vi "SignalAcqStatus.vi"(8 "error in (no error)":errorcluster caption="entrée d'erreur (pas d'erreur)", 10 "Booléen":bool=TRUE, 11 "Experiment en entrée":refnum<class "Experiment.lvclass"> caption="DNL_LabVIEW Object in") -> (0 "error out":errorcluster caption="sortie d'erreur", 3 "Experiment en sortie":refnum<class "Experiment.lvclass"> caption="DNL_LabVIEW Object out")   [LabVIEW 2019, in "Experiment.lvclass"]
uses:
  Experiment.lvclass
  Experiment.lvclass/Experiment.ctl
  <userlib>/GenProg/ArrayTo1DI32.vi
  DevicesClass/BaseDevice/BaseDevice.lvclass
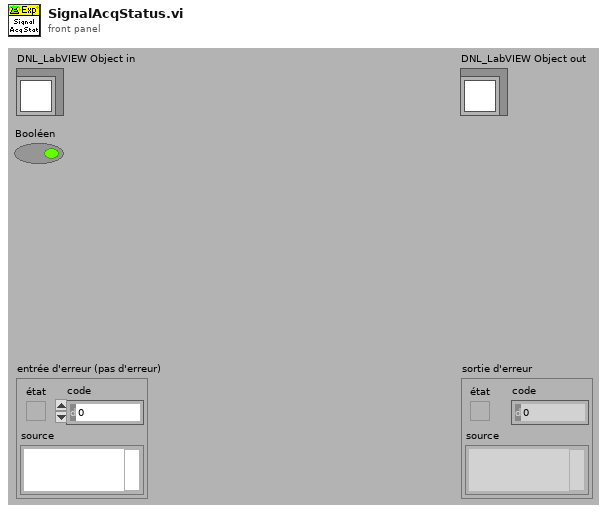
[diagram p1: front panel]
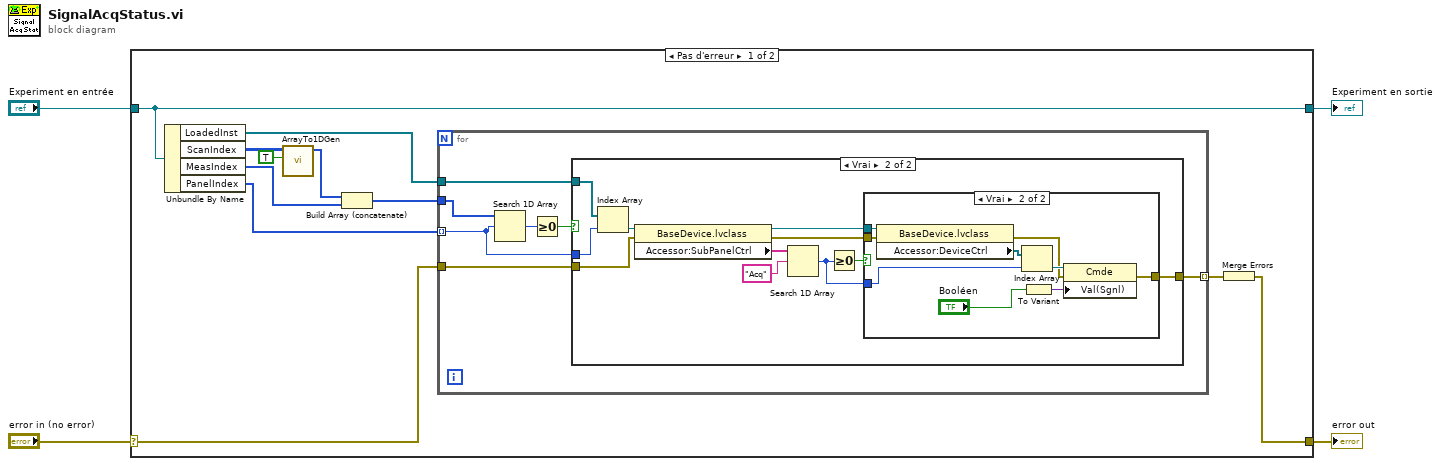
[diagram p0: block diagram]
diagram:
  n1 = case shown="Pas d'erreur" "error in (no error)" {
    selector: "error in (no error)" -> [w7 w46]
    tunnel: [w5 w46] -> w3
    tunnel: [w15 w45] -> w1
    tunnel: "Experiment en entrée" -> [w15 w45]
    frame No Error {
      n2 = Unbundle By Name(w15) -> ("LoadedInst"=w14:refnum<class "BaseDevice.lvclass">[], "ScanIndex"=w13:i32[][], "MeasIndex"=w11:i32[], "PanelIndex"=w8:i32[])
      n3 = call-poly <userlib>:"ArrayTo1DGen.vi"("DelArrEnd"=TRUE, "tableau"=w13) -> ("Array Out"=w10:i32[])  [unwired: 7 in, 2 out]
      n4 = Build Array (concatenate)(w10, w11) -> (w9:i32[])
      n5 = for {
        tunnel: w14 -> [w19]
        tunnel: w9 -> [w22]
        tunnel: w8 -> [w18] mode=indexing
        tunnel: w7 -> [w17]
        tunnel: [w16] -> w6 mode=indexing
        n6 = Search 1D Array(1D array=w22, element=w18) -> (index of element=w21:i32)  [unwired: 1 in]
        n7 = Greater Or Equal To 0?(x=w21) -> (x >= 0?=w20:bool)
        n8 = case shown="Vrai" w20 {
          tunnel: w19 -> [_ w34]
          tunnel: w18 -> [_ w33]
          tunnel: w17 -> [w23 w28]
          tunnel: [w23 w26] -> w16
          frame False {
          }
          frame True {
            n9 = Index Array(array=w34, index=w33) -> (element=w32:refnum<class "BaseDevice.lvclass">)
            n10 = property class="BaseDevice.lvclass"(reference=w32, error in=w28) -> (reference out=w29:refnum<class "BaseDevice.lvclass">, error out=w27:errorcluster, "Accessor:SubPanelCtrl"=w31:string[])
            n11 = Search 1D Array(1D array=w31, element="Acq") -> (index of element=w24:i32)  [unwired: 1 in]
            n12 = Greater Or Equal To 0?(x=w24) -> (x >= 0?=w25:bool)
            n13 = case shown="Vrai" w25 {
              tunnel: w29 -> [_ w44]
              tunnel: w27 -> [w35 w43]
              tunnel: [w35 w36] -> w26
              tunnel: w24 -> [_ w41]
              frame False {
              }
              frame True {
                n14 = property class="BaseDevice.lvclass"(reference=w44, error in=w43) -> (error out=w37:errorcluster, "Accessor:DeviceCtrl"=w42:refnum<vi>[])  [unwired: 1 out]
                n15 = Index Array(array=w42, index=w41) -> (element=w40:refnum<vi>)
                n16 = To Variant(anything="Booléen") -> (Variant=w38:variant)
                n17 = property class="Cmde"(reference=w40, error in=w37, "Val(Sgnl)"=w38) -> (error out=w36:errorcluster)  [unwired: 1 out]
              }
            }
          }
        }
      }
      n18 = Merge Errors(w6) -> (w5:errorcluster)
    }
    frame Error {
    }
  }
  "error out" <- w3
  "Experiment en sortie" <- w1
